vi "Agilent PSG MXG_Enable Output.vi"(8 "error in":errorcluster, 10 "Enable?":bool=TRUE, 11 "Handle In":variant) -> (0 "error out":errorcluster {"code" format="%.0x"}, 3 "Handle Out":variant)   [LabVIEW 2015]
uses:
  <instrlib>/Agilent PSG MXG Series/Agilent PSG MXG Series.lvlib
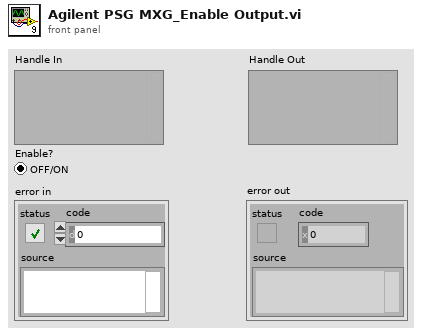
[diagram p1: front panel]
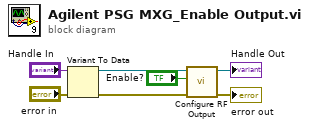
[diagram p0: block diagram]
diagram:
  n1 = Variant To Data(error in="error in", Variant="Handle In") -> (data=w1:refnum<visa-resource-name>, error out=w4:errorcluster)  [unwired: 1 in]
  n2 = call <instrlib>:"Configure RF Output.vi"("error in (no error)"=w4, "Enable RF Output (F:Disable)"="Enable?", "VISA resource name"=w1) -> ("error out"=→"error out":errorcluster, "VISA resource name out"=→"Handle Out":refnum<visa-resource-name>)  [unwired: 7 in]
